vi "Level XCtl Test.vi"() -> ()   [LabVIEW 2015]
uses:
  XControls/Level (G3)/Level Data.ctl
  XControls/Level (G3)/Level Units (G3).ctl
  XControls/Level (G3)/Level (G3).xctl
panel:
  out "Array Out":T1[](array[typedef])
  in  "Level (G3)":T3(xcontrol)
  in  "Array":T1[](array[typedef])
  in  "Apply":bool
  in  "stop":bool
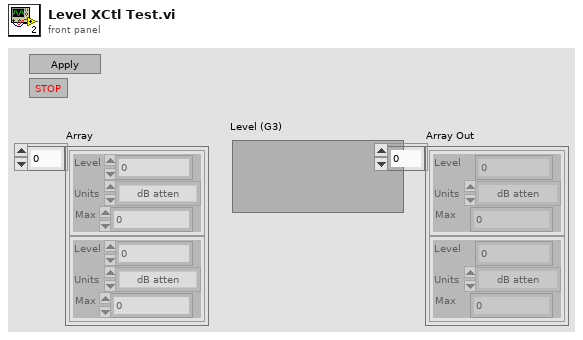
[diagram p1: front panel]
types:
  T1 = typedef "Level (G3).xctl/Level Data.ctl" = cluster{"Level":dbl, "Units":T2, "Max":dbl, "Data":cluster{"Multiplier":dbl, "Cal File":path, "Cal":cluster{"Freq (Hz)":dbl[], "Mag (dB SPL)":dbl[], "Phase (deg)":dbl[]}, "audiogram":path}}
  T2 = typedef "Level (G3).xctl/Level Units (G3).ctl" = enum16{"dB atten", "dB SPL", "dB re 1 Vrms", "dB V/Hz½", "dB SL", "mW", "Volts"}
  T3 = cluster{"Level":dbl, "Units":T2, "Max":dbl, "Data":cluster{"Multiplier":dbl, "Cal File":path, "Cal":cluster{"Freq (Hz)":dbl[], "Mag (dB SPL)":dbl[], "Phase (deg)":dbl[]}, "audiogram":path}}
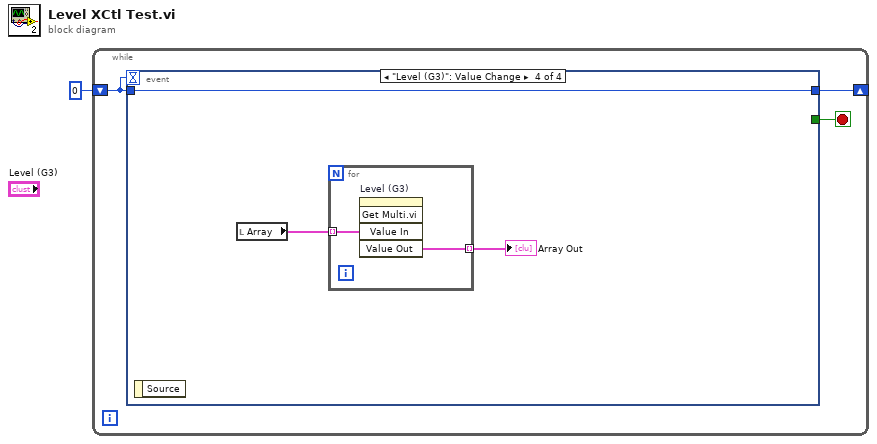
[diagram p0: block diagram]
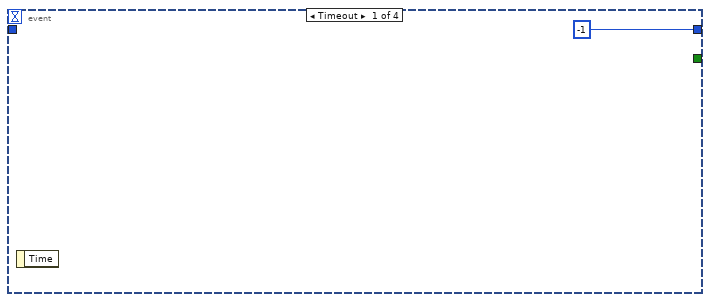
[diagram p2: hidden frame]
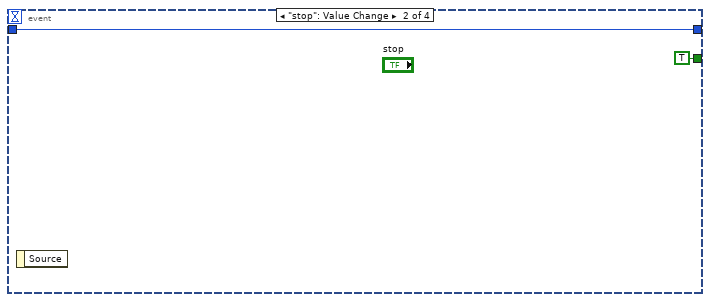
[diagram p3: hidden frame]
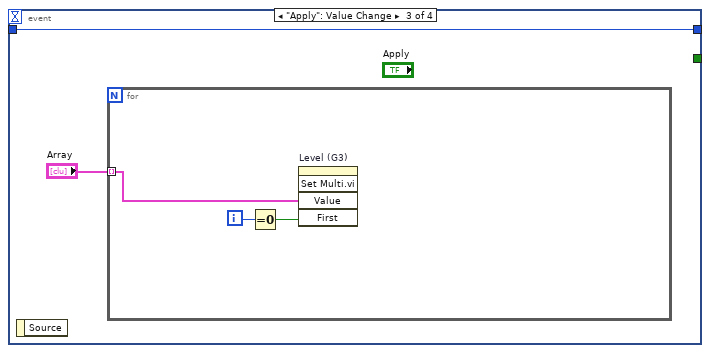
[diagram p4: hidden frame]
diagram:
  n1 = while {
    shift-right: [w2] -> _
    shift-left: 0 -> [w3]
    stop <- w4 stop-if-true
    n2 = event shown="[3] \"Level (G3)\": Value Change" {
      selector: _ -> [_ _ _ _]
      dyn-events: _ -> [_ _ _ _]
      timeout: w3 -> [_ _ _ _]
      tunnel: [_ TRUE _ _] -> w4
      tunnel: w3 -> [_ w6 w9 w15]
      tunnel: [-1 w6 w9 w15] -> w2
      event Timeout {
        n3 = event-data() -> ()  [unwired: 1 in, 1 out]
      }
      event "stop": Value Change {
        n4 = event-data() -> ()  [unwired: 1 in, 1 out]
      }
      event "Apply": Value Change {
        n5 = event-data() -> ()  [unwired: 1 in, 1 out]
        n6 = for {
          tunnel: "Array" -> [w10] mode=indexing
          i -> [w12]
          n7 = Equal To 0?(x=w12) -> (x = 0?=w11:bool)
          n8 = invoke on="Level (G3)" class="Level (G3) (strict)" method="Set Multi.vi"("Value"=w10, "First"=w11) -> ()  [unwired: 3 in, 5 out]
        }
      }
      event "Level (G3)": Value Change {
        n9 = event-data() -> ()  [unwired: 1 in, 1 out]
        n10 = local read "Array"() -> (w14:T1[])
        n11 = for {
          tunnel: w14 -> [w17] mode=indexing
          tunnel: [w16] -> w13 mode=indexing
          n12 = invoke on="Level (G3)" class="Level (G3) (strict)" method="Get Multi.vi"("Value In"=w17) -> ("Value Out"=w16:T1)  [unwired: 4 in, 4 out]
        }
        "Array Out" <- w13
      }
    }
  }
